vi "Inverse_Kinematics.vi"(4 "B3":dbl[](array[numeric]), 5 "px":dbl, 6 "pz":dbl, 7 "B2":dbl[](array[numeric]), 8 "py":dbl, 9 "B1":dbl[](array[numeric])) -> (0 "Reset Inputs":bool, 1 "theta 3":dbl, 2 "theta 2":dbl, 3 "theta 1":dbl)   [LabVIEW 2016]
doc: "This VI converts the desired tool tip position (px,py,pz) into joint motions of theta 1, theta 2, and theta 3.\nB1, B2, and B3 are 2-element arrays containing lower and upper bounds for joint motions.\n\"Reset Inputs\" sends out a boolean value (T) if an error occurs."
panel:
  out "Err Msg":bool
  out "theta 1 UB":dbl
  out "theta 1 LB":dbl
  out "theta 2 UB":dbl
  out "theta 2 LB":dbl
  out "theta 3 UB":dbl
  out "theta 3 LB":dbl
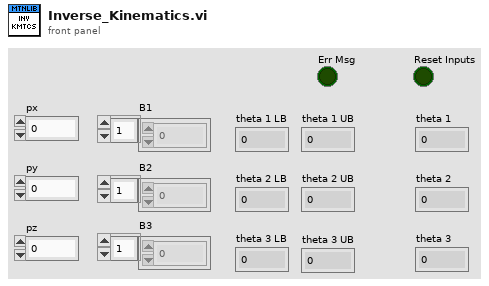
[diagram p1: front panel]
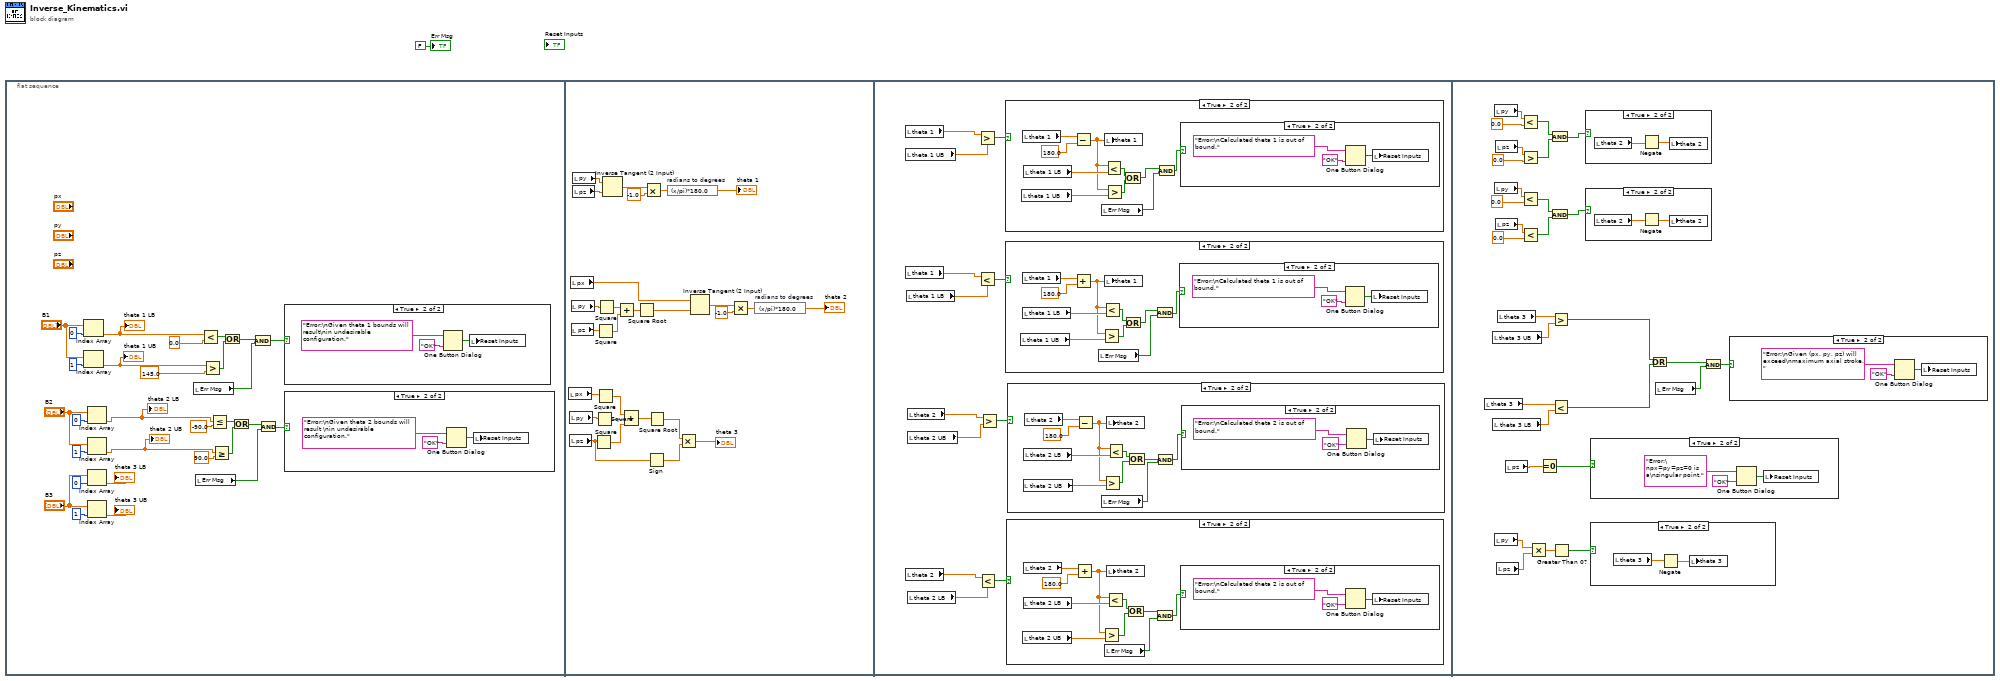
[diagram p0: block diagram]
diagram:
  n1 = flat-sequence {
    frame #0 {
      n2 = Index Array(array="B1", index=0) -> (element=w9:dbl)
      "theta 1 LB" <- w9
      n3 = Index Array(array="B1", index=1) -> (element=w8:dbl)
      "theta 1 UB" <- w8
      n4 = Index Array(array="B2", index=0) -> (element=w13:dbl)
      "theta 2 LB" <- w13
      n5 = Index Array(array="B2", index=1) -> (element=w10:dbl)
      "theta 2 UB" <- w10
      n6 = Index Array(array="B3", index=0) -> (element=→"theta 3 LB":dbl)
      n7 = Index Array(array="B3", index=1) -> (element=→"theta 3 UB":dbl)
      n8 = local read "Err Msg"() -> (w3:bool)
      n9 = local read "Err Msg"() -> (w2:bool)
      n10 = Less?(x=w9, y=0.0) -> (x < y?=w21:bool)
      n11 = Greater?(x=w8, y=145.0) -> (0:w18:bool)
      n12 = Less Or Equal?(x=w13, y=-90.0) -> (x <= y?=w14:bool)
      n13 = Greater Or Equal?(x=w10, y=90.0) -> (x >= y?=w17:bool)
      n14 = Or(x=w21, y=w18) -> (x .or. y?=w7:bool)
      n15 = Or(x=w14, y=w17) -> (x .or. y?=w4:bool)
      n16 = And(x=w7, y=w3) -> (x .and. y?=w6:bool)
      n17 = And(x=w4, y=w2) -> (x .and. y?=w5:bool)
      n18 = case shown="True" w6 {
        frame False {
        }
        frame True {
          n19 = One Button Dialog(message="Error:\nGiven theta 1 bounds will result\nin undesirable configuration.", button name ("OK")="OK" ("F button name (\"Cancel\")")) -> (true=w34:bool)
          n20 = local write "Reset Inputs"(w34) -> ()
        }
      }
      n21 = case shown="True" w5 {
        frame False {
        }
        frame True {
          n22 = One Button Dialog(message="Error:\nGiven theta 2 bounds will result \nin undesirable configuration.", button name ("OK")="OK" ("F button name (\"Cancel\")")) -> (true=w31:bool)
          n23 = local write "Reset Inputs"(w31) -> ()
        }
      }
    }
    frame #1 {
      n24 = local read "px"() -> (w59:dbl)
      n25 = local read "py"() -> (w58:dbl)
      n26 = local read "pz"() -> (w40:dbl)
      n27 = local read "px"() -> (w51:dbl)
      n28 = local read "py"() -> (w52:dbl)
      n29 = local read "pz"() -> (w53:dbl)
      n30 = local read "py"() -> (w41:dbl)
      n31 = local read "pz"() -> (w42:dbl)
      n32 = Square(x=w40) -> (x^2=w62:dbl)
      n33 = Square(x=w58) -> (x^2=w61:dbl)
      n34 = Square(x=w59) -> (x^2=w60:dbl)
      n35 = Square(x=w53) -> (x^2=w55:dbl)
      n36 = Square(x=w52) -> (x^2=w54:dbl)
      n37 = Inverse Tangent (2 Input)(1:w42, 2:w41) -> (0:w43:dbl)
      n38 = Add(x=w54, y=w55) -> (x+y=w56:dbl)
      n39 = Compound Arithmetic op=ADD(w60, w61, w62) -> (w63:dbl)
      n40 = Square Root(x=w56) -> (sqrt(x)=w57:dbl)
      n41 = Multiply(x=w43, y=sgl -1.0) -> (x*y=w45:dbl)
      n42 = Sign(1:w40) -> (0:w38:dbl)
      n43 = Square Root(x=w63) -> (sqrt(x)=w39:dbl)
      n44 = expression code="(x/pi)*180.0" "radians to degrees"(w45) -> (→"theta 1":dbl)
      n45 = Multiply(x=w39, y=w38) -> (x*y=→"theta 3":dbl)
      n46 = Inverse Tangent (2 Input)(1:w57, 2:w51) -> (0:w50:dbl)
      n47 = Multiply(x=w50, y=sgl -1.0) -> (x*y=w48:dbl)
      n48 = expression code="(x/pi)*180.0" "radians to degrees"(w48) -> (→"theta 2":dbl)
    }
    frame #2 {
      n49 = local read "theta 1"() -> (w65:dbl)
      n50 = local read "theta 1"() -> (w68:dbl)
      n51 = local read "theta 1 UB"() -> (w66:dbl)
      n52 = local read "theta 2"() -> (w71:dbl)
      n53 = local read "theta 1 LB"() -> (w67:dbl)
      n54 = local read "theta 2"() -> (w74:dbl)
      n55 = local read "theta 2 LB"() -> (w72:dbl)
      n56 = local read "theta 2 UB"() -> (w73:dbl)
      n57 = Greater?(x=w65, y=w66) -> (0:w64:bool)
      n58 = Less?(x=w68, y=w67) -> (x < y?=w69:bool)
      n59 = Less?(x=w71, y=w72) -> (x < y?=w70:bool)
      n60 = Greater?(x=w74, y=w73) -> (0:w75:bool)
      n61 = case shown="True" w64 {
        frame False {
        }
        frame True {
          n62 = local read "theta 1 UB"() -> (w118:dbl)
          n63 = local read "theta 1"() -> (w124:dbl)
          n64 = local read "theta 1 LB"() -> (w122:dbl)
          n65 = Subtract(x=w124, y=180.0) -> (x-y=w119:dbl)
          n66 = local read "Err Msg"() -> (w120:bool)
          n67 = Less?(x=w119, y=w122) -> (x < y?=w117:bool)
          n68 = local write "theta 1"(w119) -> ()
          n69 = Greater?(x=w119, y=w118) -> (0:w116:bool)
          n70 = Compound Arithmetic op=OR(w117, w116) -> (w115:bool)
          n71 = And(x=w115, y=w120) -> (x .and. y?=w121:bool)
          n72 = case shown="True" w121 {
            frame False {
            }
            frame True {
              n73 = One Button Dialog(message="Error:\nCalculated theta 1 is out of bound.", button name ("OK")="OK" ("F button name (\"Cancel\")")) -> (true=w127:bool)
              n74 = local write "Reset Inputs"(w127) -> ()
            }
          }
        }
      }
      n75 = case shown="True" w69 {
        frame False {
        }
        frame True {
          n76 = local read "theta 1 UB"() -> (w105:dbl)
          n77 = local read "theta 1"() -> (w111:dbl)
          n78 = local read "theta 1 LB"() -> (w109:dbl)
          n79 = Add(x=w111, y=180.0) -> (x+y=w104:dbl)
          n80 = local read "Err Msg"() -> (w107:bool)
          n81 = Greater?(x=w104, y=w105) -> (0:w106:bool)
          n82 = Less?(x=w104, y=w109) -> (x < y?=w103:bool)
          n83 = local write "theta 1"(w104) -> ()
          n84 = Compound Arithmetic op=OR(w103, w106) -> (w102:bool)
          n85 = And(x=w102, y=w107) -> (x .and. y?=w108:bool)
          n86 = case shown="True" w108 {
            frame False {
            }
            frame True {
              n87 = One Button Dialog(message="Error:\nCalculated theta 1 is out of bound.", button name ("OK")="OK" ("F button name (\"Cancel\")")) -> (true=w114:bool)
              n88 = local write "Reset Inputs"(w114) -> ()
            }
          }
        }
      }
      n89 = case shown="True" w70 {
        frame False {
        }
        frame True {
          n90 = local read "theta 2 UB"() -> (w80:dbl)
          n91 = local read "theta 2 LB"() -> (w83:dbl)
          n92 = local read "theta 2"() -> (w85:dbl)
          n93 = Add(x=w85, y=180.0) -> (x+y=w79:dbl)
          n94 = Greater?(x=w79, y=w80) -> (0:w77:bool)
          n95 = local read "Err Msg"() -> (w81:bool)
          n96 = Less?(x=w79, y=w83) -> (x < y?=w78:bool)
          n97 = local write "theta 2"(w79) -> ()
          n98 = Compound Arithmetic op=OR(w78, w77) -> (w76:bool)
          n99 = And(x=w76, y=w81) -> (x .and. y?=w82:bool)
          n100 = case shown="True" w82 {
            frame False {
            }
            frame True {
              n101 = One Button Dialog(message="Error:\nCalculated theta 2 is out of bound.", button name ("OK")="OK" ("F button name (\"Cancel\")")) -> (true=w88:bool)
              n102 = local write "Reset Inputs"(w88) -> ()
            }
          }
        }
      }
      n103 = case shown="True" w75 {
        frame False {
        }
        frame True {
          n104 = local read "theta 2 UB"() -> (w92:dbl)
          n105 = local read "theta 2 LB"() -> (w96:dbl)
          n106 = local read "theta 2"() -> (w98:dbl)
          n107 = Subtract(x=w98, y=180.0) -> (x-y=w93:dbl)
          n108 = local read "Err Msg"() -> (w89:bool)
          n109 = Greater?(x=w93, y=w92) -> (0:w91:bool)
          n110 = Less?(x=w93, y=w96) -> (x < y?=w94:bool)
          n111 = local write "theta 2"(w93) -> ()
          n112 = Compound Arithmetic op=OR(w94, w91) -> (w90:bool)
          n113 = And(x=w90, y=w89) -> (x .and. y?=w95:bool)
          n114 = case shown="True" w95 {
            frame False {
            }
            frame True {
              n115 = One Button Dialog(message="Error:\nCalculated theta 2 is out of bound.", button name ("OK")="OK" ("F button name (\"Cancel\")")) -> (true=w101:bool)
              n116 = local write "Reset Inputs"(w101) -> ()
            }
          }
        }
      }
    }
    frame #3 {
      n117 = local read "theta 3"() -> (w130:dbl)
      n118 = local read "theta 3 UB"() -> (w154:dbl)
      n119 = local read "theta 3 LB"() -> (w155:dbl)
      n120 = local read "py"() -> (w134:dbl)
      n121 = local read "py"() -> (w151:dbl)
      n122 = local read "py"() -> (w137:dbl)
      n123 = local read "pz"() -> (w147:dbl)
      n124 = local read "pz"() -> (w138:dbl)
      n125 = local read "pz"() -> (w133:dbl)
      n126 = local read "theta 3"() -> (w153:dbl)
      n127 = local read "pz"() -> (w156:dbl)
      n128 = Less?(x=w151, y=0.0) -> (x < y?=w145:bool)
      n129 = Less?(x=w137, y=0.0) -> (x < y?=w140:bool)
      n130 = Greater?(x=w147, y=0.0) -> (0:w144:bool)
      n131 = Less?(x=w138, y=0.0) -> (x < y?=w141:bool)
      n132 = Multiply(x=w134, y=w133) -> (x*y=w132:dbl)
      n133 = Equal To 0?(x=w156) -> (x = 0?=w135:bool)
      n134 = And(x=w145, y=w144) -> (x .and. y?=w143:bool)
      n135 = And(x=w140, y=w141) -> (x .and. y?=w142:bool)
      n136 = Greater?(x=w153, y=w154) -> (0:w129:bool)
      n137 = Less?(x=w130, y=w155) -> (x < y?=w128:bool)
      n138 = Greater Than 0?(x=w132) -> (x > 0?=w131:bool)
      n139 = case shown="True" w143 {
        frame False {
        }
        frame True {
          n140 = local read "theta 2"() -> (w168:dbl)
          n141 = Negate(x=w168) -> (-x=w167:dbl)
          n142 = local write "theta 2"(w167) -> ()
        }
      }
      n143 = case shown="True" w142 {
        frame False {
        }
        frame True {
          n144 = local read "theta 2"() -> (w160:dbl)
          n145 = Negate(x=w160) -> (-x=w159:dbl)
          n146 = local write "theta 2"(w159) -> ()
        }
      }
      n147 = case shown="True" w135 {
        frame False {
        }
        frame True {
          n148 = One Button Dialog(message="Error:\npx=py=pz=0 is a\nsingular point.", button name ("OK")="OK" ("F button name (\"Cancel\")")) -> (true=w161:bool)
          n149 = local write "Reset Inputs"(w161) -> ()
        }
      }
      n150 = case shown="True" w131 {
        frame False {
        }
        frame True {
          n151 = local read "theta 3"() -> (w158:dbl)
          n152 = Negate(x=w158) -> (-x=w157:dbl)
          n153 = local write "theta 3"(w157) -> ()
        }
      }
      n154 = Or(x=w129, y=w128) -> (x .or. y?=w150:bool)
      n155 = local read "Err Msg"() -> (w148:bool)
      n156 = And(x=w150, y=w148) -> (x .and. y?=w149:bool)
      n157 = case shown="True" w149 {
        frame False {
        }
        frame True {
          n158 = One Button Dialog(message="Error:\nGiven (px, py, pz) will exceed\nmaximum axial stroke.", button name ("OK")="OK" ("F button name (\"Cancel\")")) -> (true=w166:bool)
          n159 = local write "Reset Inputs"(w166) -> ()
        }
      }
    }
  }
  "Err Msg" <- FALSE ("Err Msg")
